vi "Get Last.vi"(0 "Conditional Branch in":refnum<class "Conditional Branch.lvclass">, 1 "Linked List Ref":refnum<data-value>, 5 "Active Unique ID":string, 9 "Active Element Index":i32, 11 "error in (no error)":errorcluster) -> (3 "Linked List Ref out":refnum<data-value>, 4 "Executioner out":refnum<class "Executioner.lvclass">, 6 "Active Unique ID out":string, 10 "Active Element Index out":i32, 12 "Restore Point":bool, 13 "Complete":bool, 14 "Stop":bool, 15 "error out":errorcluster)   [LabVIEW 2017, in "Test Executive.lvlib" / "Conditional Branch.lvclass"]
uses:
  <vilib>/gpm_packages/@cs/test-executive/Source/Test Executive/Conditional Branch/Conditional Branch.lvclass
  C:/Program Files/National Instruments/LabVIEW 2017/vi.lib/gpm_packages/@cs/test-executive/Source/Test Executive/Executioner/Executioner.lvclass
  <vilib>/gpm_packages/@cs/test-executive/Source/Test Executive/Executioner/Executioner.lvclass
  <vilib>/gpm_packages/@cs/linked-list/Source/Linked List/ILinkedList/ILinked List.lvclass
  fa23959a-2204-4e23-9b96-24d9ce150fe4.vi
  <vilib>/gpm_packages/@cs/linked-list/Source/Linked List/Linked List Ref/Linked List Ref.lvclass
  5b7e822d-91b0-4ac7-aaa1-f549dbb63cea.vi
  e1a69301-650a-4345-9450-f58f2c381fc0.vi
  f0edb87c-4e86-49af-8722-aeda4b938978.vi
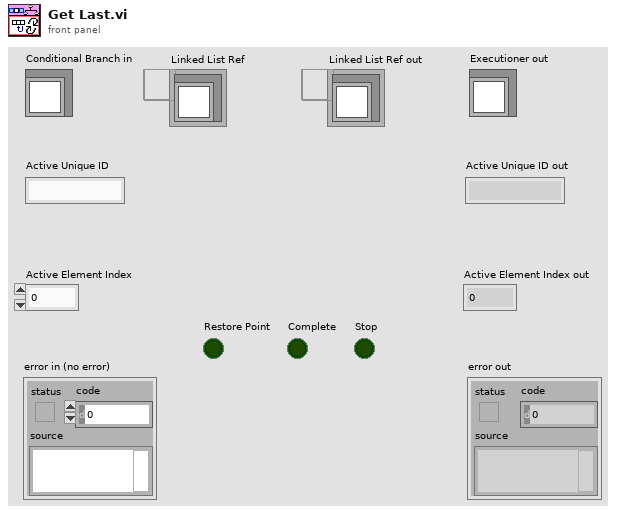
[diagram p1: front panel]
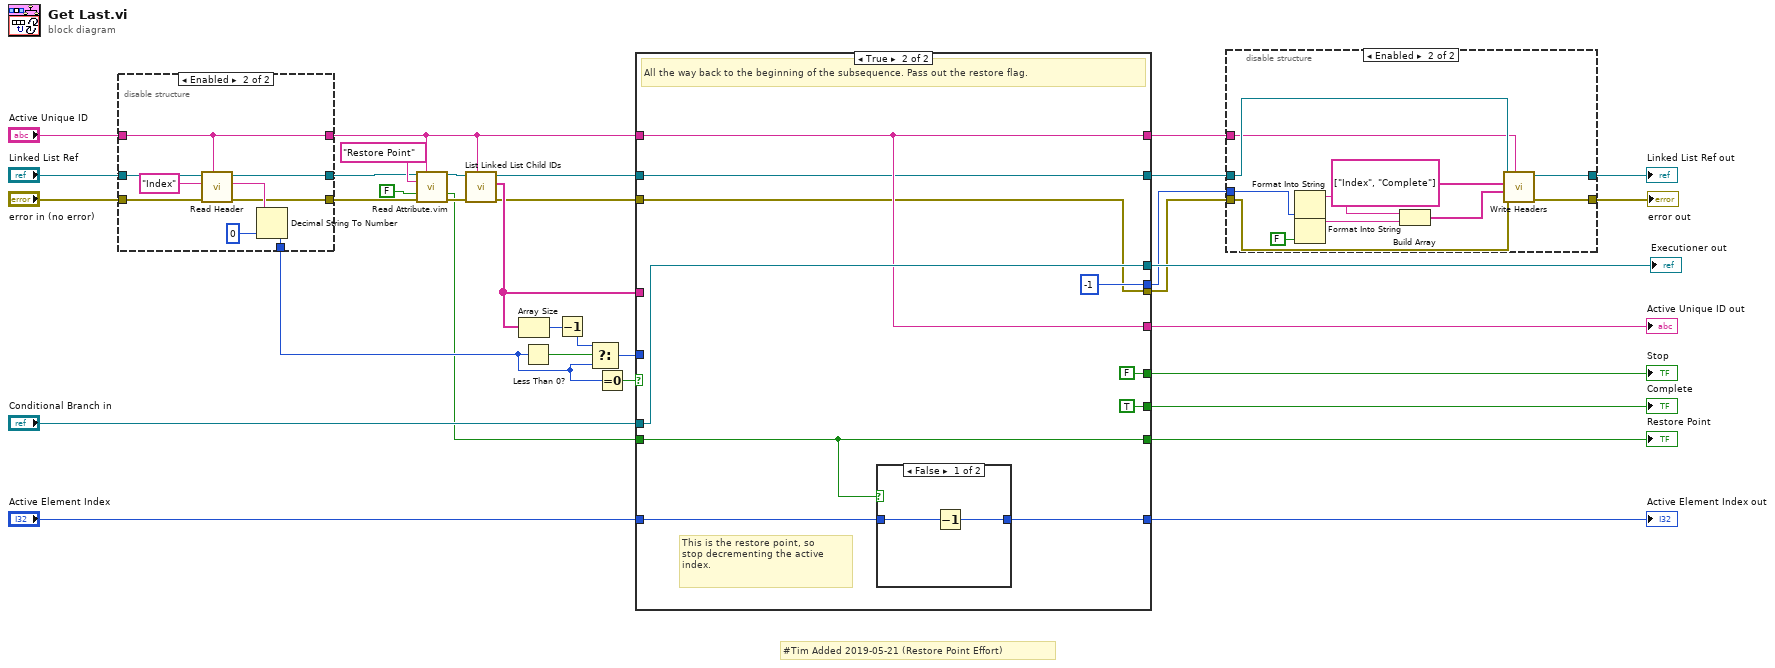
[diagram p0: block diagram]
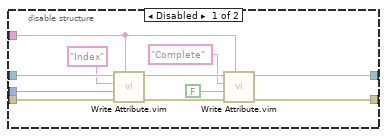
[diagram p2: hidden frame]
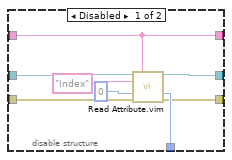
[diagram p3: hidden frame]
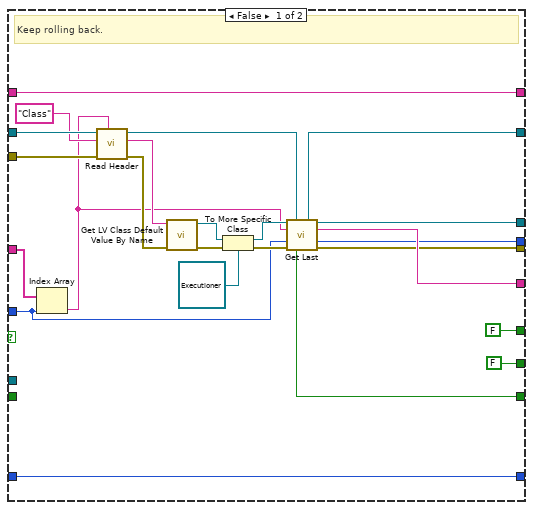
[diagram p4: hidden frame]
diagram:
  # "#Tim Added 2019-05-21 (Restore Point Effort)"
  n1 = disable-structure shown="Enabled" {
    disable-tunnel: "Linked List Ref" -> [w42 w48]
    disable-tunnel: "error in (no error)" -> [w39 w46]
    disable-tunnel: [w38 w45] -> w22
    disable-tunnel: "Active Unique ID" -> [w35 w43]
    disable-tunnel: [w37 w47] -> w4
    disable-tunnel: [w36 w44] -> w3
    disable-tunnel: [w35 w43] -> w1
    frame Disabled {
      n2 = call "Read Attribute.vim"("Linked List Ref"=w42, "Linked List ID"=w35, "Attribute Name"="Index", "Type"=0, "error in (no error)"=w39) -> ("Linked List Ref out"=w37:refnum<data-value>, "Attribute"=w38:i32, "error out"=w36:errorcluster)  [unwired: 5 in, 3 out]
    }
    frame Enabled {
      n3 = call <vilib>:"Read Header.vi"("Linked List ID"=w43, "error in (no error)"=w46, "Header Name"="Index" ("Attribute Name"), "Linked List Ref"=w48) -> ("error out"=w44:errorcluster, "Header Value"=w50:string, "Linked List Ref out"=w47:refnum<data-value>)  [unwired: 4 in, 1 out]
      n4 = Decimal String To Number(string=w50, default (0L)=0 ("Attribute")) -> (number=w45:i32)  [unwired: 1 in, 1 out]
    }
  }
  n5 = call "Read Attribute.vim"("Linked List Ref"=w4, "Linked List ID"=w1, "Attribute Name"="Restore Point", "Type"=FALSE, "error in (no error)"=w3) -> ("Linked List Ref out"=w29:refnum<data-value>, "Attribute"=w2:bool, "error out"=w30:errorcluster)  [unwired: 5 in, 3 out]
  n6 = call <vilib>:"List Linked List Child IDs.vi"("Linked List ID"=w1, "error in (no error)"=w30, "Linked List Ref"=w29) -> ("error out"=w20:errorcluster, "Child IDs"=w21:string[], "Linked List Ref out"=w28:refnum<data-value>)  [unwired: 6 in]
  n7 = Array Size(array=w21) -> (size(s)=w27:i32)
  n8 = Less Than 0?(x=w22) -> (x < 0?=w26:bool)
  n9 = Decrement(x=w27) -> (x-1=w25:i32)
  n10 = Select(t=w25, s=w26, f=w22) -> (s? t:f=w24:i32)
  n11 = Equal To 0?(x=w22) -> (x = 0?=w23:bool)
  n12 = case shown="True" w23 {
    tunnel: w28 -> [w74 w78]
    tunnel: w24 -> [w65 _]
    tunnel: w21 -> [w75 _]
    tunnel: w20 -> [w72 w77]
    tunnel: "Active Element Index" -> [w64 w81]
    tunnel: [w64 w80] -> w18
    tunnel: "Conditional Branch in" -> [_ w84]
    tunnel: [w62 w78] -> w10
    tunnel: [w59 w79] -> w16
    tunnel: [w58 w84] -> w15
    tunnel: w1 -> [w57 w79]
    tunnel: [w57 w79] -> w9
    tunnel: [w56 w77] -> w8
    tunnel: [w55 w76] -> w11
    tunnel: [w54 -1 ("Active Element Index out")] -> w7
    tunnel: [FALSE ("Complete") TRUE ("Complete")] -> w6
    tunnel: [FALSE ("Complete") FALSE ("Complete")] -> w5
    tunnel: w2 -> [_ w76]
    frame False {
      # "Keep rolling back."
      n13 = Index Array(array=w75, index=w65) -> (element=w60:string)
      n14 = call <vilib>:"Read Header.vi"("Linked List ID"=w60, "error in (no error)"=w72, "Header Name"="Class", "Linked List Ref"=w74) -> ("error out"=w70:errorcluster, "Header Value"=w71:string, "Linked List Ref out"=w63:refnum<data-value>)  [unwired: 4 in, 1 out]
      n15 = call <vilib>:"Get LV Class Default Value By Name.vi"("error in (no error)"=w70, "class name"=w71) -> ("error out"=w69:errorcluster, "object"=w68:refnum<class>)  [unwired: 8 in]
      n16 = To More Specific Class(target class=refnum<class "Executioner.lvclass"> refnum ("Test Executive.lvlib:Executioner.lvclass"), reference=w68, error in=w69) -> (specific class reference=w61:refnum<class "Executioner.lvclass">, error out=w66:errorcluster)
      n17 = call-dynamic "Get Last.vi"("Executioner in"=w61, "Linked List Ref"=w63, "Active Unique ID"=w60, "Active Element Index"=w65, "error in (no error)"=w66) -> ("Linked List Ref out"=w62:refnum<data-value>, "Executioner out"=w58:refnum<class "Executioner.lvclass">, "Active Unique ID out"=w59:string, "Active Element Index out"=w54:i32, "Restore Point"=w55:bool, "error out"=w56:errorcluster)  [unwired: 3 in, 2 out]
    }
    frame True {
      # "This is the restore point, so\nstop decrementing the active\nindex."
      # "All the way back to the beginning of the subsequence. Pass out the restore flag."
      n18 = case shown="False" w76 {
        tunnel: w81 -> [w87 w88]
        tunnel: [w86 w88] -> w80
        frame False {
          n19 = Decrement(x=w87) -> (x-1=w86:i32)
        }
        frame True {
        }
      }
    }
  }
  "Executioner out" <- w15
  "Active Unique ID out" <- w16
  "Active Element Index out" <- w18
  "Restore Point" <- w11
  "Complete" <- w6
  "Stop" <- w5
  n20 = disable-structure shown="Enabled" {
    disable-tunnel: [w99 w105] -> w14
    disable-tunnel: [w98 w102] -> w13
    disable-tunnel: w10 -> [w97 w106]
    disable-tunnel: w9 -> [w95 w104]
    disable-tunnel: w8 -> [w93 w103]
    disable-tunnel: w7 -> [w92 w101]
    frame Disabled {
      n21 = call "Write Attribute.vim"("Linked List ID"=w95, "error in (no error)"=w93, "Attribute"=w92, "Attribute Name"="Index", "Linked List Ref"=w97) -> ("error out"=w90:errorcluster, "Linked List Ref out"=w96:refnum<data-value>)  [unwired: 3 in, 2 out]
      n22 = call "Write Attribute.vim"("Linked List ID"=w95, "error in (no error)"=w90, "Attribute"=FALSE ("Complete"), "Attribute Name"="Complete", "Linked List Ref"=w96) -> ("error out"=w98:errorcluster, "Linked List Ref out"=w99:refnum<data-value>)  [unwired: 3 in, 2 out]
    }
    frame Enabled {
      n23 = Format Into String(w101) -> (resulting string=w109:string)  [unwired: 3 in, 1 out]
      n24 = Format Into String(FALSE ("input 1")) -> (resulting string=w108:string)  [unwired: 3 in, 1 out]
      n25 = Build Array(w109, w108) -> (w107:string[])
      n26 = call <vilib>:"Write Headers.vi"("Linked List ID"=w104, "error in (no error)"=w103, "Header Values"=w107, "Header Names"=string[] ["Index", "Complete"], "Linked List Ref"=w106) -> ("error out"=w102:errorcluster, "Linked List Ref out"=w105:refnum<data-value>)  [unwired: 5 in]
    }
  }
  "error out" <- w13
  "Linked List Ref out" <- w14
